vi "Configure Display Number Format.vi"(8 "error in (no error)":errorcluster, 10 "format":u16(ring) items=["floating point", "exponential"], 11 "VGC in":refnum<class "PL Inficon VGC.lvclass">) -> (0 "error out":errorcluster, 2 "format":u16(ring) items=["floating point", "exponential"], 3 "VGC out":refnum<class "PL Inficon VGC.lvclass">)   [LabVIEW 2015, in "PL Inficon VGC.lvclass"]
doc: "Configures display number format."
uses:
  PL Inficon VGC.lvclass
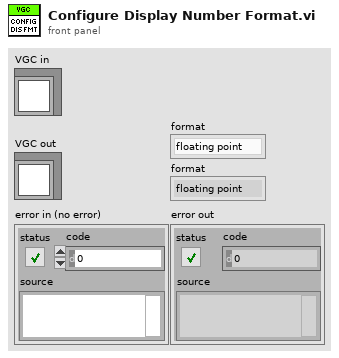
[diagram p1: front panel]
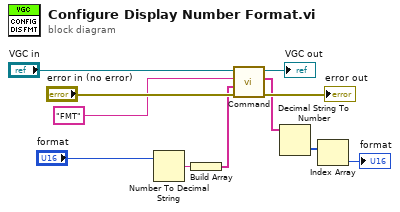
[diagram p0: block diagram]
diagram:
  n1 = Number To Decimal String(number="format") -> (decimal integer string=w4:string)  [unwired: 1 in]
  n2 = Build Array(w4) -> (w2:string[])
  n3 = call "Command.vi"("error in (no error)"="error in (no error)", "parameters"=w2, "command"="FMT" ("format string"), "VGC in"="VGC in") -> ("error out"=→"error out":errorcluster, "response data"=w6:string[], "VGC out"=→"VGC out":refnum<class "PL Inficon VGC.lvclass">)  [unwired: 5 in]
  n4 = Decimal String To Number(string=w6) -> (number=w7:i32[])  [unwired: 2 in, 1 out]
  n5 = Index Array(array=w7) -> (element=→"format":i32)  [unwired: 1 in]
